vi "OpenConnection.vi"(8 "error in (no error)":errorcluster, 11 "RSeries_CAM in":refnum<class "RSeries_CAM.lvclass">) -> (0 "error out":errorcluster, 3 "RSeries_CAM out":refnum<class "RSeries_CAM.lvclass">)   [LabVIEW 2024, in "RSeries_CAM.lvlib" / "RSeries_CAM.lvclass"]
uses:
  RSeries_CAM.lvclass
  RSeries_CAM.lvclass/RSeries_CAM.ctl
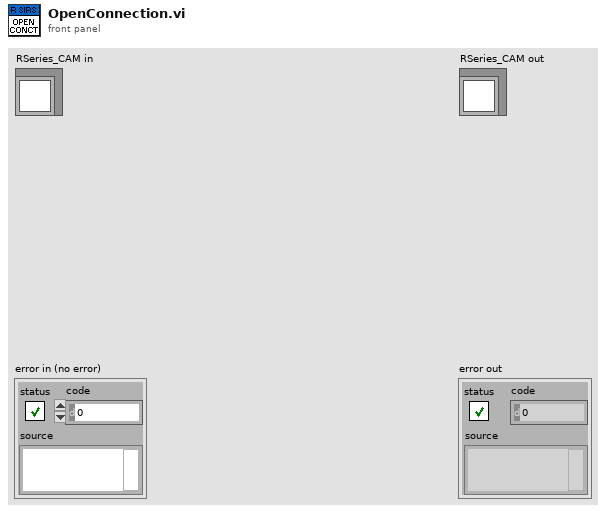
[diagram p1: front panel]
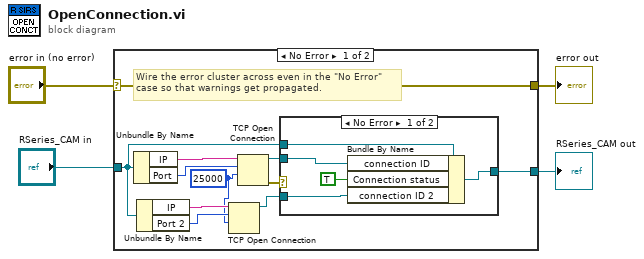
[diagram p0: block diagram]
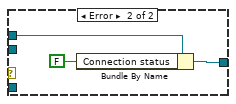
[diagram p2: hidden frame]
diagram:
  n1 = case shown="No Error" "error in (no error)" {
    selector: "error in (no error)" -> [w15 w25]
    tunnel: [w15 w25] -> w3
    tunnel: [w10 w24] -> w1
    tunnel: "RSeries_CAM in" -> [w9 w24]
    frame No Error {
      w5 = 25000 ("timeout ms (60000)")
      # "Wire the error cluster across even in the \"No Error\"\ncase so that warnings get propagated."
      n2 = Unbundle By Name(w9) -> ("IP"=w14:string, "Port"=w13:u32)
      n3 = Unbundle By Name(w9) -> ("IP"=w8:string, "Port 2"=w7:u32)
      n4 = TCP Open Connection(address=w8, remote port or service name=w7, timeout ms (60000)=w5) -> (connection ID=w6:refnum<k5>)  [unwired: 2 in, 1 out]
      n5 = TCP Open Connection(address=w14, remote port or service name=w13, timeout ms (60000)=w5) -> (connection ID=w11:refnum<k5>, error out=w12:errorcluster)  [unwired: 2 in]
      n6 = case shown="No Error" w12 {
        tunnel: w9 -> [w20 w23]
        tunnel: w11 -> [w19 _]
        tunnel: [w17 w21] -> w10
        tunnel: w6 -> [w16 _]
        frame No Error {
          n7 = Bundle By Name(cluster=w20, "connection ID"=w19, "Connection status"=TRUE, "connection ID 2"=w16) -> (w17:refnum<class "RSeries_CAM.lvclass">)
        }
        frame Error {
          n8 = Bundle By Name(cluster=w23, "Connection status"=FALSE) -> (w21:refnum<class "RSeries_CAM.lvclass">)
        }
      }
    }
    frame Error {
    }
  }
  "error out" <- w3
  "RSeries_CAM out" <- w1
